vi "Convert Tree Data and Save to XML.vi"(7 "tag":string[](array[string]), 8 "error in":errorcluster, 9 "Value":string[](array[string]), 10 "Step":string[](array[string]), 11 "file":path) -> (0 "error out":errorcluster, 2 "StepObj Out":refnum<class "STEP.lvclass">[](array[class]), 3 "path":path)   [LabVIEW 2015]
uses:
  Reusable/Sequence/STEPS/STEP.lvclass
  <vilib>/xml/Close Reference(Node).vi
  <resource>/objmgr/DOMUserDefRef.rc
  <vilib>/xml/NI_XML.lvlib
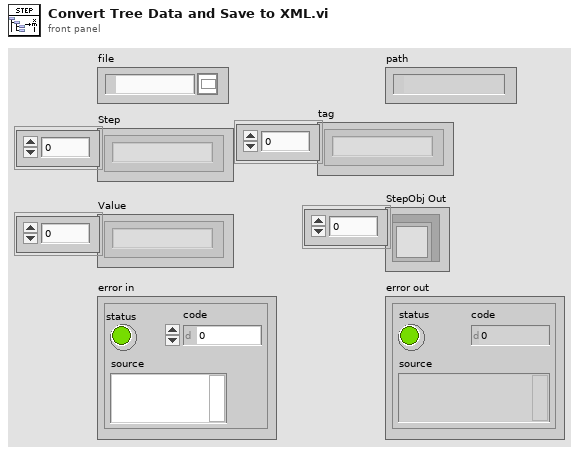
[diagram p1: front panel]
types:
  T1 = enum16{"open", "replace", "create", "open or create", "replace or create", "replace or create with confirmation"}
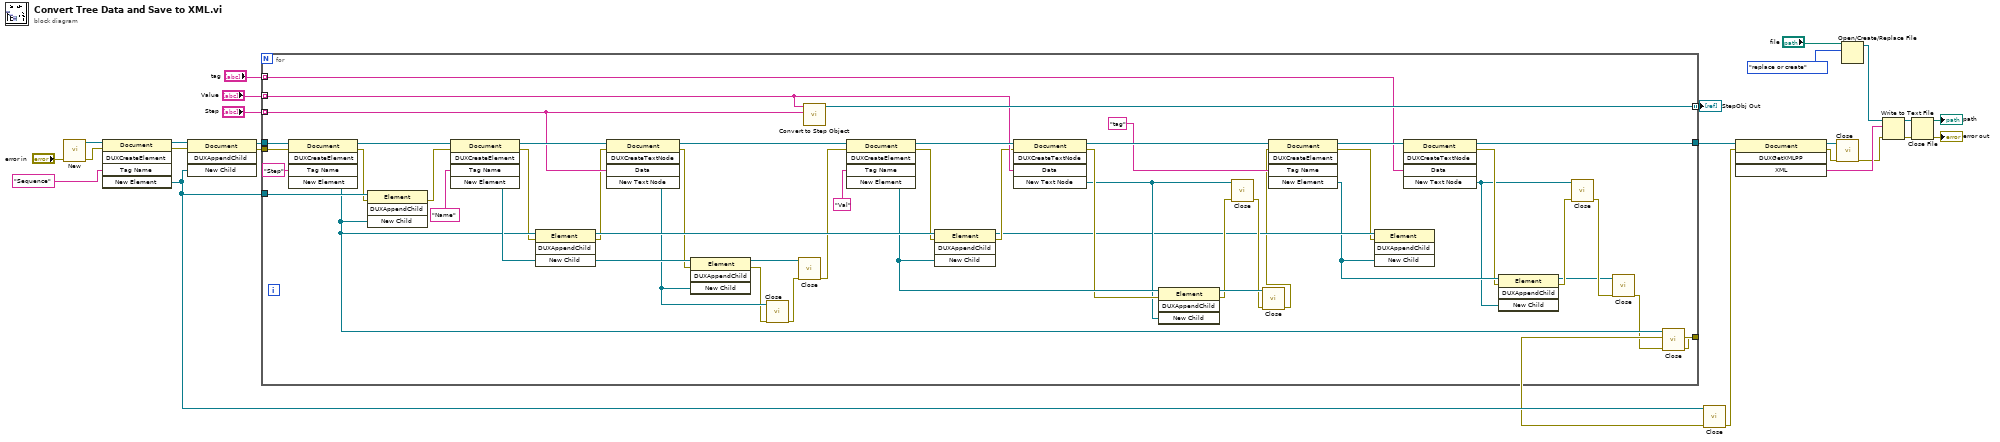
[diagram p0: block diagram]
diagram:
  n1 = call <vilib>:"New.vi"("error in (no error)"="error in") -> ("error out"=w13:errorcluster, "DOM document out"=w12:refnum<k20>)  [unwired: 7 out]
  n2 = invoke class="Document" method="DUXCreateElement"(reference=w12, error in=w13, "Tag Name"="Sequence" ("Qualified Name")) -> (reference out=w15:refnum<k20>, error out=w21:errorcluster, "New Element"=w23:refnum<k20>)  [unwired: 2 in, 2 out]
  n3 = invoke class="Document" method="DUXAppendChild"(reference=w15, error in=w21, "New Child"=w23) -> (reference out=w16:refnum<k20>, error out=w22:errorcluster)  [unwired: 1 in, 2 out]
  n4 = for {
    tunnel: "Step" -> [w70] mode=indexing
    tunnel: "Value" -> [w63] mode=indexing
    tunnel: [w77] -> w27 mode=indexing
    tunnel: w16 -> [w76]
    tunnel: w23 -> [w74]
    tunnel: [w59] -> w17
    tunnel: w22 -> [w43]
    tunnel: [w28] -> w24
    tunnel: "tag" -> [w37] mode=indexing
    n5 = invoke class="Document" method="DUXCreateElement"(reference=w76, error in=w43, "Tag Name"="Step") -> (reference out=w72:refnum<k20>, error out=w48:errorcluster, "New Element"=w60:refnum<k20>)  [unwired: 2 in, 2 out]
    n6 = invoke class="Element" method="DUXAppendChild"(reference=w74, error in=w48, "New Child"=w60) -> (error out=w47:errorcluster)  [unwired: 1 in, 3 out]
    n7 = invoke class="Document" method="DUXCreateElement"(reference=w72, error in=w47, "Tag Name"="Name") -> (reference out=w71:refnum<k20>, error out=w46:errorcluster, "New Element"=w69:refnum<k20>)  [unwired: 2 in, 2 out]
    n8 = invoke class="Element" method="DUXAppendChild"(reference=w60, error in=w46, "New Child"=w69) -> (reference out=w65:refnum<k20>, error out=w45:errorcluster)  [unwired: 1 in, 2 out]
    n9 = invoke class="Document" method="DUXCreateTextNode"(reference=w71, error in=w45, "Data"=w70) -> (reference out=w66:refnum<k20>, error out=w44:errorcluster, "New Text Node"=w58:refnum<k20>)  [unwired: 2 in, 2 out]
    n10 = invoke class="Element" method="DUXAppendChild"(reference=w69, error in=w44, "New Child"=w58) -> (reference out=w68:refnum<k20>, error out=w57:errorcluster)  [unwired: 1 in, 2 out]
    n11 = call-poly <vilib>:"Close.vi"("error in (no error)"=w57, "node"=w58) -> ("error out"=w56:errorcluster)  [unwired: 7 out]
    n12 = call-poly <vilib>:"Close.vi"("error in (no error)"=w56, "node"=w68) -> ("error out"=w55:errorcluster)  [unwired: 7 out]
    n13 = call "Convert to Step Object.vi"("Step"=w70, "Value"=w63) -> ("STEP out"=w77:refnum<class "STEP.lvclass">)  [unwired: 8 in, 1 out]
    n14 = invoke class="Document" method="DUXCreateElement"(reference=w66, error in=w55, "Tag Name"="Val") -> (reference out=w64:refnum<k20>, error out=w54:errorcluster, "New Element"=w62:refnum<k20>)  [unwired: 2 in, 2 out]
    n15 = invoke class="Element" method="DUXAppendChild"(reference=w65, error in=w54, "New Child"=w62) -> (reference out=w40:refnum<k20>, error out=w53:errorcluster)  [unwired: 1 in, 2 out]
    n16 = invoke class="Document" method="DUXCreateTextNode"(reference=w64, error in=w53, "Data"=w63) -> (reference out=w42:refnum<k20>, error out=w52:errorcluster, "New Text Node"=w51:refnum<k20>)  [unwired: 2 in, 2 out]
    n17 = invoke class="Element" method="DUXAppendChild"(reference=w62, error in=w52, "New Child"=w51) -> (reference out=w61:refnum<k20>, error out=w50:errorcluster)  [unwired: 1 in, 2 out]
    n18 = call-poly <vilib>:"Close.vi"("error in (no error)"=w50, "node"=w51) -> ("error out"=w49:errorcluster)  [unwired: 7 out]
    n19 = call-poly <vilib>:"Close.vi"("error in (no error)"=w49, "node"=w61) -> ("error out"=w30:errorcluster)  [unwired: 7 out]
    n20 = invoke class="Document" method="DUXCreateElement"(reference=w42, error in=w30, "Tag Name"="tag" ("Data")) -> (reference out=w38:refnum<k20>, error out=w39:errorcluster, "New Element"=w36:refnum<k20>)  [unwired: 2 in, 2 out]
    n21 = invoke class="Element" method="DUXAppendChild"(reference=w40, error in=w39, "New Child"=w36) -> ()  [unwired: 1 in, 4 out]
    n22 = invoke class="Document" method="DUXCreateTextNode"(reference=w38, "Data"=w37) -> (reference out=w28:refnum<k20>, error out=w35:errorcluster, "New Text Node"=w34:refnum<k20>)  [unwired: 3 in, 2 out]
    n23 = invoke class="Element" method="DUXAppendChild"(reference=w36, error in=w35, "New Child"=w34) -> (reference out=w31:refnum<k20>, error out=w33:errorcluster)  [unwired: 1 in, 2 out]
    n24 = call-poly <vilib>:"Close.vi"("error in (no error)"=w33, "node"=w34) -> ("error out"=w32:errorcluster)  [unwired: 7 out]
    n25 = call-poly <vilib>:"Close.vi"("error in (no error)"=w32, "node"=w31) -> ("error out"=w29:errorcluster)  [unwired: 7 out]
    n26 = call-poly <vilib>:"Close.vi"("error in (no error)"=w29, "node"=w60) -> ("error out"=w59:errorcluster)  [unwired: 7 out]
  }
  "StepObj Out" <- w27
  n27 = call-poly <vilib>:"Close.vi"("error in (no error)"=w17, "node"=w23) -> ("error out"=w20:errorcluster)  [unwired: 7 out]
  n28 = invoke class="Document" method="DUXGetXMLPP"(reference=w24, error in=w20) -> (reference out=w19:refnum<k20>, error out=w18:errorcluster, "XML"=w25:string)  [unwired: 2 in, 1 out]
  n29 = call-poly <vilib>:"Close.vi"("error in (no error)"=w18, "node"=w19) -> ("error out"=w8:errorcluster)  [unwired: 7 out]
  n30 = Open/Create/Replace File(file path (use dialog)="file", operation (0:open)=T1."replace or create") -> (refnum out=w2:refnum<file>)  [unwired: 4 in, 2 out]
  n31 = Write to Text File(file (use dialog)=w2, text=w25, error in=w8) -> (refnum out=w26:refnum<file>, error out=w7:errorcluster)  [unwired: 1 in, 1 out]
  n32 = Close File(refnum=w26, error in=w7) -> (path=→"path":path, error out=→"error out":errorcluster)
